vi "FPGA Main High Throughput.vi"() -> ()   [LabVIEW 2019]
doc: "The myRIO v1.2 FPGA Shipping Personality. This personality contains support for:\n- 1 Button\n- 4 LED\n- 4 Analog Input channels with 1 Sample\n- 1 Analog Input channel with N Samples\n- 2 Analog Output channels with 1 Sample\n- 1 Analog Output channel with N Samples\n- 16 Digital I/O channels with 1 Sample\n- 1 Digital Input channel with N Samples\n- 1 Digital Output channel with N Samples"
uses:
  Sub VIs/Utilities/Start Boolean.ctl
  <vilib>/Platform/TimedLoop/XDataNode/timing_clust.ctl
  <vilib>/Platform/TimedLoop/XDataNode/nitl_modes.ctl
  <vilib>/Platform/TimedLoop/XDataNode/wakeup.ctl
  <vilib>/rvi/Emulation/niFpgaGetClockAttributes.vi
  <vilib>/rvi/Emulation/niFpgaSctlEmulationGetInTimedLoop.vi
  <vilib>/rvi/Emulation/niFpgaEmulationReportErrorSimple.vi
  <vilib>/rvi/eio/common/nirviEmuTemplateMethod_errors.vi
  <vilib>/rvi/Emulation/niFpgaProcessEmulError.vi
  <vilib>/rvi/Emulation/niFpgaCriticalErrorInLSC.vi
  <vilib>/rvi/Emulation/niFpgaEmulationIsFPGAContextNoSignature.vi
  <vilib>/rvi/errors/niFpgaSetErrorForExecOnDevCompSimple.vi
  <vilib>/rvi/eio/common/nirviEmuReportErrorAndStop.vi
  <vilib>/rvi/DataTransferAndStorage/Container/Common/niFpgaContainerGetUniqueNameForEmu.vi
  <vilib>/rvi/FIFO/Fifo_Resource/nirvififoEmulationSetSize.vi
  <vilib>/rvi/FIFO/Fifo_Resource/nirviFifoEmulationQueueMgr.vi
  <instcachedir>/0/nirviFifoEmulationQueueMgr_E5CAEC123FF24DC58D834DCA3CDAA9B5.lvgen/nirviFifoEmulationQueueMgr_E5CAEC123FF24DC58D834DCA3CDAA9B5_002.vi
  <vilib>/Utility/error.llb/Clear Errors.vi
  <vilib>/rvi/FIFO/Fifo_Resource/nirvififoEmulationCreateLock.vi
  <vilib>/rvi/FIFO/Fifo_Resource/nirvififoEmulationObtainLock.vi
  <vilib>/rvi/FIFO/Fifo_Resource/nirvififoEmulationReleaseLock.vi
  <vilib>/rvi/occurrence/nirviWaitOnOccurrenceBase.vi
  <vilib>/rvi/errors/nirviReportUnexpectedCaseInternalError.vi
  <vilib>/rvi/errors/nirviReportUnexpectedCaseInternalError (U32).vi
  <vilib>/rvi/FIFO/Fifo_Resource/nirvififoEmulationDetermineInputValidOut.vi
  <vilib>/rvi/interface/RandomDataEmulation/niFpgaRandomDataHandleErrors.vi
  <vilib>/rvi/DataTransferAndStorage/Container/Common/niFpgaContainerSetEmuInfo.vi
  <vilib>/rvi/DataTransferAndStorage/Container/Common/niFpgaContainerExecOnDevCompGetState.vi
  <vilib>/eio/EIONode/EIONode.xnode
  <vilib>/rvi/DataTransferAndStorage/Container/XNode/niFpgaContainer.xnode
  <vilib>/rvi/FIFO/Fifo_Resource/nirvififoEmulationRead.vi
  <vilib>/rvi/FIFO/Fifo_Resource/nirvififoEmulationWrite.vi
  <vilib>/rvi/interface/RandomDataEmulation/nirviRandomDataFpgaReadWriteTemplate.vi
  <vilib>/Platform/TimedLoop/XDataNode/XDataNode.xnode
  <vilib>/rvi/LocalResourceManager/LocalResourceManager.xnode
  <vilib>/rvi/FIFO/Fifo_Resource/niFpgaFifoEmulationRefIn.vi
  <vilib>/Platform/TimedLoop/XDataNode/XDNodeRunTimeDep.lvlib
panel:
  out "AI.B_1.VAL":u16
  out "AI.B_2.VAL":u16
  out "AI.B_3.VAL":u16
  out "AI.B_0.VAL":u16
  in  "AO.B_1.VAL":u16
  in  "AO.B_0.VAL":u16
  out "DIO.B_7:0.IN":u8 format="%08b"
  in  "DIO.B_7:0.DIR":u8 format="%08b"
  in  "DIO.B_7:0.OUT":u8 format="%08b"
  in  "SYS.SELECTB":u8 format="%08b"
  out "DIO.B_15:8.IN":u8 format="%08b"
  in  "DIO.B_15:8.DIR":u8 format="%08b"
  in  "DIO.B_15:8.OUT":u8 format="%08b"
  in  "DO.A_1.IRQ.SELECT":bool
  in  "AO.A_0.IRQ.SELECT":bool
  in  "AO.A_0.VAL":u16
  out "AO.A_0.IDL":bool
  out "AO.SYS.STAT":bool
  in  "AO.SYS.GO":T1
  in  "AO.A_1.VAL":u16
  out "AI.A_0.VAL":u16
  out "AI.A_3.VAL":u16
  out "AI.A_2.VAL":u16
  out "AI.A_1.VAL":u16
  in  "DO.A_1.ClockDivisor":u16 caption="AO LoopRate(Ticks)"
  in  "DI.A_0.ClockDivisor":u16 caption="AO LoopRate(Ticks)"
  out "DO.A_1.IDL":bool
  in  "DI.A_0.ENA":bool
  out "DI.A_0.IDL":bool
  out "DIO.A_15:8.IN":u8 format="%08b"
  in  "DIO.A_15:8.DIR":u8 format="%08b"
  in  "DIO.A_15:8.OUT":u8 format="%08b"
  out "DIO.A_7:0.IN":u8 format="%08b"
  in  "DIO.A_7:0.DIR":u8 format="%08b"
  in  "DIO.A_7:0.OUT":u8 format="%08b"
  out "AI.A_0.IDL":bool
  in  "AI.A_0.SampleRate":u32=40000 caption="Count(Ticks)"
  out "SYS.AI.RDY":bool
  in  "AO.A_0.SampleRate":u32=40000 caption="AO LoopRate(Ticks)"
  out "SYS.RDY":bool
  out "SYS.BLOCK.A/AI0.RDY":bool
  in  "SYS.SELECTA":u8 format="%08b"
  out "DI.BTN":u8 format="%08b"
  in  "DO.LED3:0":u8 format="%04b"
  out "ACC.X.VAL":u16
  out "ACC.Y.VAL":u16
  out "SYS.ACC.RDY":bool
  out "ACC.Z.VAL":u16
  # "System"
  # "Connector B"
  # "Connector A"
  # "Onboard Devices"
  # "Accelerometer"
  # "Analog Input"
  # "Analog Output"
  # "Digital I/O"
  # "Analog Input"
  # "Analog Output"
  # "Digital I/O"
  # "Block Write AO"
  # "Buttons & LEDs"
  # "IO Configuration"
  # "Block Read AI"
  # "Block Read DI"
  # "Block Write DO"
  # "IO Configuration"
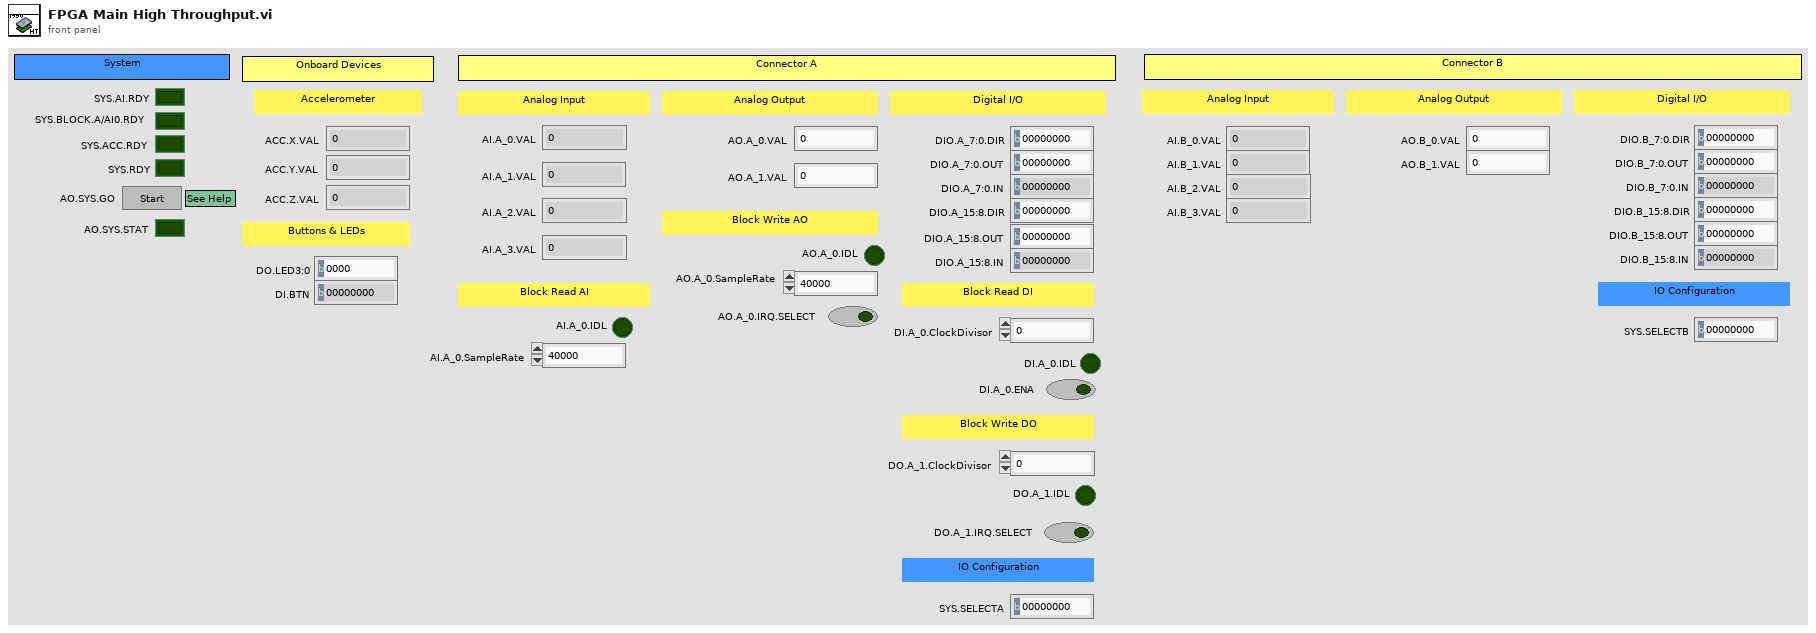
[diagram p1: front panel]
types:
  T1 = typedef "Start Boolean.ctl" = bool
  T2 = typedef "XDNodeRunTimeDep.lvlib/timing_clust.ctl" = cluster{"Expected End [f-1]":u64, "Actual End [f-1]":u64, "Finished Late? [f-1]":bool, "Expected End [i-1]":u64, "Actual End [i-1]":u64, "Finished Late? [i-1]":bool, "Expected Start [i]":u64, "Actual Start [i]":u64, "Expected Start [f]":u64, "Actual Start [f]":u64, "Source Name":string, "Structure Name":string, "Period":i64, "Deadline":i64, "Offset":i64, "Start":i64, "Priority":i32, "Timeout":i32, "Mode":T3, "Wakeup Reason":T4, "Error":errorcluster, "Source Type":string, "Secondary Source Type":string, "Global End Time":u64, "Global Start Time":u64, "Frame Duration":u64, "Iteration Duration":u64, "Assigned CPU":i32, "I/O Scan Engine Mode":u32}
  T3 = typedef "XDNodeRunTimeDep.lvlib/nitl_modes.ctl" = enum32{"No Change", "Process missed periods, maintain original phase", "Discard missed periods, maintain original phase", "Process missed periods, ignore original phase", "Discard missed periods, ignore original phase"}
  T4 = typedef "XDNodeRunTimeDep.lvlib/wakeup.ctl" = enum32{"Normal", "Aborted", "Asynchronous wakeup", "Timing source error", "Timed loop error", "Timeout"}
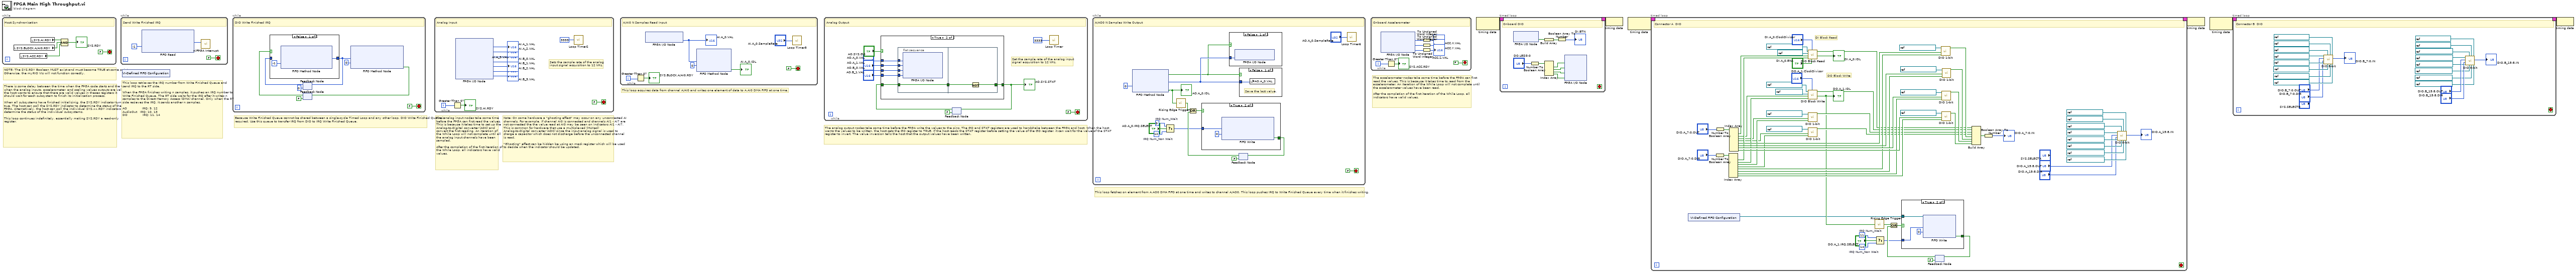
[diagram p0: block diagram]
diagram:
  # "This loop acquires data from channel A/AI0 and writes one element of data to A.AI0 DMA FIFO at one time."
  # "The accelerometer nodes take some time before the FPGA can first read the values. This is because it takes time to read from the accelerometer. An iteration of the While Loop will not complete until the accelerometer values have been read.\n\nAfter the completion of the first iteration of the While Loop, all indicators have valid values."
  # "This loop fetches on element from A.AO0 DMA FIFO at one time and writes to channel A/AO0. This loop pushes IRQ to Write Finished Queue every time when it finishes writing."
  # "The analog output nodes take some time before the FPGA write the values to the pins. The GO and STAT registers are used to handshake between the FPGA and host. When the host wants the values to be written, the host sets the GO register to TRUE. If the host reads the STAT register before setting the value of the GO register, it can wait for the value of the STAT register to invert. The value inversion tells the host that the output values have been written."
  # "The analog input nodes take some time before the FPGA can first read the values. This is because it takes time to set up the Analog-to-Digital converter (ADC) and convert the first reading. An iteration of the While Loop will not complete until all the analog input channels have been sampled.\n\nAfter the completion of the first iteration of the While Loop, all indicators have valid values."
  # "Because Write Finished Queue cannot be shared between a single-cycle Timed Loop and any other loop, DIO Write Finished Queue is required. Use this queue to transfer IRQ from DIO to IRQ Write Finished Queue."
  # "This loop retrieves the IRQ number from Write Finished Queue and send IRQ to the RT side. \n\nWhen the FPGA finishes writing n samples, it pushes an IRQ number to Write Finished Queue. The RT side waits for the IRQ after it writes n samples to the Direct Memory Access (DMA) channel. Only when the RT side recieves the IRQ, it sends another n samples.\n\nAO               IRQ: 9, 12\nAudioOut   IRQ: 10, 13\nDO               IRQ: 11, 14"
  # "NOTE: The SYS.RDY Boolean MUST exist and must become TRUE at some point. Otherwise, the myRIO VIs will not function correctly."
  # "There is some delay between the time when the FPGA code starts and the time when the analog inputs, accelerometer, and scaling values outputs are valid. If the host wants to ensure that there are valid values in theses registers it should wait for each subsystem to finish its initialization process. \n\nWhen all subsystems have finished initializinig, the SYS.RDY indicator turns true. The host can poll the SYS.RDY indicator to determine the status of the FPGA. Alternatively, the host can poll the individual SYS.xx.RDY indicators to determine the status of the individual subsystems.\n\nThis loop continues indefinitely, essentially making SYS.RDY a read-only register."
  # "Note: On some hardware a \"ghosting effect\" may occur on any unconnected AI channels. For example, if channel AI0 is connected and channels AI1 - AI7 are not connected the the value read at AI0 may be seen on indicators AI1 - AI7. This is common for hardware that use a multiplexed (MUXed) Analog-to-Digital converter (ADC) since the input analog signal is used to charge a capacitor which does not discharge before the unconnected channel is read.\n\n\"Ghosting\" effect can be hidden be using an mask register which will be used to decide when the indicator should be updated."
  n1 = while {
    stop <- FALSE stop-if-true
    # "Host Synchronization"
    n2 = local read "SYS.BLOCK.A/AI0.RDY"() -> (w9:bool)
    n3 = local read "SYS.ACC.RDY"() -> (w7:bool)
    n4 = local read "SYS.AI.RDY"() -> (w11:bool)
    n5 = Compound Arithmetic op=AND(w11, w9, w7) -> (→"SYS.RDY":bool)
  }
  n6 = while {
    stop <- FALSE stop-if-true
    # "Send Write Finished IRQ"
    n7 = xnode ("FIFO Read")("Timeout"=-1) -> ("Element"=w14:u8)  [unwired: 1 in, 2 out]
    n8 = call <vilib>:"niFPGA Interrupt.vi"("IRQ Number (0)"=w14) -> ()  [unwired: 2 in]
  }
  n9 = xnode "VI-Defined FIFO Configuration"() -> ()  [unwired: 1 out]
  n10 = while {
    stop <- FALSE stop-if-true
    # "DIO Write Finished IRQ"
    n11 = feedback #1(u8 0 ("Element")) -> (w17:u8)
    n12 = feedback #2(FALSE ("Timed Out?")) -> (w21:bool)
    n13 = case shown="False" w21 {
      tunnel: [w23 w25] -> w18
      tunnel: w17 -> [_ w25]
      frame False {
        n14 = xnode ("FIFO Method Node")("Timeout"=-1) -> ("Element"=w23:u8)  [unwired: 1 in, 2 out]
      }
      frame True {
      }
    }
    n15 = feedback-in #1(w18) -> ()
    n16 = xnode ("FIFO Method Node")("Element"=w18, "Timeout"=0) -> ("Timed Out?"=w19:bool)  [unwired: 1 in, 1 out]
    n17 = feedback-in #2(w19) -> ()
  }
  n18 = while {
    i -> [w30]
    stop <- FALSE stop-if-true
    # "Sets the sample rate of the analog \ninput signal acquisition to 12 kHz."
    # "Analog Input"
    n19 = Greater Than 0?(x=w30) -> (x > 0?=→"SYS.AI.RDY":bool)
    n20 = xnode "FPGA I/O Node"() -> ("ConnectorA/AI1"=→"AI.A_1.VAL":u16, "ConnectorA/AI2"=→"AI.A_2.VAL":u16, "ConnectorA/AI3"=→"AI.A_3.VAL":u16, "ConnectorB/AI0"=→"AI.B_0.VAL":u16, "ConnectorB/AI1"=→"AI.B_1.VAL":u16, "ConnectorB/AI2"=→"AI.B_2.VAL":u16, "ConnectorB/AI3"=→"AI.B_3.VAL":u16)  [unwired: 7 in, 7 out]
    n21 = call "Loop Timer2"("Count(Ticks)"=u32 3333) -> ()  [unwired: 1 out]
  }
  n22 = while {
    i -> [w38]
    stop <- FALSE stop-if-true
    # "A/AI0 N Samples Read Input"
    n23 = Greater Than 0?(x=w38) -> (x > 0?=→"SYS.BLOCK.A/AI0.RDY":bool)
    n24 = xnode "FPGA I/O Node"() -> ("ConnectorA/AI0"=w39:u16)  [unwired: 1 in, 1 out]
    "AI.A_0.VAL" <- w39
    n25 = xnode ("FIFO Method Node")("Element"=w39, "Timeout"=0) -> ("Timed Out?"=→"AI.A_0.IDL":bool)  [unwired: 1 in, 1 out]
    n26 = call "Loop Timer5"("Count(Ticks)"="AI.A_0.SampleRate") -> ()  [unwired: 1 out]
  }
  n27 = while {
    stop <- FALSE stop-if-true
    # "Set the sample rate of the analog input \nsignal acquisition to 12 kHz."
    # "Analog Output"
    n28 = feedback #3(FALSE) -> (w50:bool)
    n29 = case shown="True" "AO.SYS.GO" {
      tunnel: "AO.A_0.VAL" -> [_ w61]
      tunnel: "AO.A_1.VAL" -> [_ w60]
      tunnel: w50 -> [w54 w59]
      tunnel: [w54 w57] -> w49
      tunnel: "AO.B_0.VAL" -> [_ w56]
      tunnel: "AO.B_1.VAL" -> [_ w55]
      frame False {
      }
      frame True {
        n30 = flat-sequence {
          tunnel: w61 -> [w66]
          tunnel: w60 -> [w65]
          tunnel: w59 -> [w64]
          tunnel: [w64] -> w58
          tunnel: w56 -> [w63]
          tunnel: w55 -> [w62]
          tunnel: w58 -> [w68]
          tunnel: [w67] -> w57
          frame #0 {
            n31 = xnode "FPGA I/O Node"("ConnectorA/AO0"=w66, "ConnectorA/AO1"=w65, "ConnectorB/AO0"=w63, "ConnectorB/AO1"=w62) -> ()  [unwired: 4 in, 4 out]
          }
          frame #1 {
            n32 = Not(x=w68) -> (.not. x?=w67:bool)
          }
        }
      }
    }
    "AO.SYS.STAT" <- w49
    n33 = feedback-in #3(w49) -> ()
    n34 = call "Loop Timer"("Count(Ticks)"=u32 3333) -> ()  [unwired: 1 out]
  }
  n35 = while {
    stop <- FALSE stop-if-true
    w72 = u8 12  # IRQ Num_Non Wait
    w70 = u8 9  # IRQ Num_Wait
    # "A/AO0 N Samples Write Output"
    n36 = xnode ("FIFO Method Node")("Timeout"=0) -> ("Element"=w80:u16, "Timed Out?"=w78:bool)  [unwired: 1 in, 1 out]
    "AO.A_0.IDL" <- w78
    n37 = Select(t=w70, s="AO.A_0.IRQ.SELECT", f=w72) -> (s? t:f=w69:u8)
    n38 = call "Rising Edge Trigger.vi"("Signal"=w78) -> ("Trigger?"=w73:bool)
    n39 = case shown="False" w78 {
      tunnel: w80 -> [w87 _]
      frame False {
        n40 = xnode "FPGA I/O Node"("ConnectorA/AO0"=w87) -> ()  [unwired: 1 in, 1 out]
      }
      frame True {
      }
    }
    n41 = feedback #4(FALSE ("Timed Out?")) -> (w74:bool)
    n42 = Or(x=w73, y=w74) -> (x .or. y?=w76:bool)
    n43 = case shown="True" w76 {
      selector: w76 -> [w83 _]
      tunnel: [w83 w86] -> w75
      tunnel: w69 -> [_ w84]
      frame False {
      }
      frame True {
        n44 = xnode ("FIFO Write")("Element"=w84, "Timeout"=0) -> ("Timed Out?"=w86:bool)  [unwired: 1 in, 1 out]
      }
    }
    n45 = feedback-in #4(w75) -> ()
    n46 = case shown="False" w78 {
      tunnel: w80 -> [w88 _]
      frame False {
        # "Save the last value."
        n47 = local write "AO.A_0.VAL"(w88) -> ()
      }
      frame True {
      }
    }
    n48 = call "Loop Timer6"("Count(Ticks)"="AO.A_0.SampleRate") -> ()  [unwired: 1 out]
  }
  n49 = while {
    i -> [w93]
    stop <- FALSE stop-if-true
    # "Onboard Accelerometer"
    n50 = xnode "FPGA I/O Node"() -> ("AccelerationX"=w96:i16, "AccelerationY"=w95:i16, "AccelerationZ"=w94:i16)  [unwired: 3 in, 3 out]
    n51 = Greater Than 0?(x=w93) -> (x > 0?=→"SYS.ACC.RDY":bool)
    n52 = To Unsigned Word Integer(number=w96) -> (unsigned 16bit integer=→"ACC.X.VAL":u16)
    n53 = To Unsigned Word Integer(number=w95) -> (unsigned 16bit integer=→"ACC.Y.VAL":u16)
    n54 = To Unsigned Word Integer(number=w94) -> (unsigned 16bit integer=→"ACC.Z.VAL":u16)
  }
  n55 = node-c288() -> (w4:T2)  [unwired: 1 in]
  n56 = timed-loop {
    timing: w4 -> [_]
    timing-out: [_] -> w3
    stop <- _ stop-if-true
    # "Onboard DIO"
    n57 = xnode "FPGA I/O Node"() -> ("Button0"=w106:bool)  [unwired: 1 in, 1 out]
    n58 = Number To Boolean Array(number="DO.LED3:0") -> (Boolean array=w102:bool[])
    n59 = Build Array(w106) -> (w105:bool[])
    n60 = Index Array(array=w102) -> (element #1=w101:bool, element #2=w100:bool, element #3=w99:bool, element #4=w98:bool)  [unwired: 4 in]
    n61 = Boolean Array To Number(Boolean array=w105) -> (number=→"DI.BTN":u8)
    n62 = xnode "FPGA I/O Node"("LED0"=w101, "LED1"=w100, "LED2"=w99, "LED3"=w98) -> ()  [unwired: 4 in, 4 out]
  }
  n63 = node-c288(w3) -> ()
  n64 = node-c288() -> (w6:T2)  [unwired: 1 in]
  n65 = timed-loop {
    timing: w6 -> [_]
    timing-out: [_] -> w5
    stop <- _ stop-if-true
    w112 = u8 14  # IRQ Num_Non Wait
    w113 = u8 11  # IRQ Num_Wait
    # "DO Block Write"
    # "DI Block Read"
    # "Connector A  DIO"
    n66 = xnode "VI-Defined FIFO Configuration"() -> ("FIFO Out"=w109:refnum<k21>)
    n67 = Number To Boolean Array(number="DIO.A_7:0.DIR") -> (Boolean array=w154:bool[])
    n68 = Number To Boolean Array(number="DIO.A_7:0.OUT") -> (Boolean array=w160:bool[])
    n69 = Index Array(array=w154) -> (element #1=w137:bool, element #2=w135:bool, element #3=w132:bool, element #4=w130:bool, element #5=w153:bool, element #6=w152:bool, element #7=w151:bool, element #8=w150:bool)  [unwired: 8 in]
    n70 = Index Array(array=w160) -> (element #1=w139:bool, element #2=w136:bool, element #3=w133:bool, element #4=w131:bool, element #5=w158:bool, element #6=w157:bool, element #7=w156:bool, element #8=w155:bool)  [unwired: 8 in]
    n71 = call "DIO 1-bit.vi"("DIR"=w132, "OUT"=w133, "DIO Refnum"=refnum<k21> "ConnectorA/DIO2") -> ("IN"=w129:bool)  [unwired: 8 in]
    n72 = call "DIO Block Read.vi"("ENA"="DI.A_0.ENA", "Divisor"="DI.A_0.ClockDivisor", "DIR"=w137, "OUT"=w139, "FIFO In"=refnum<k21> "A.DI0 DMA", "DIO Refnum"=refnum<k21> "ConnectorA/DIO0" ("DIO.0/QE.A")) -> ("Timed Out?"=→"DI.A_0.IDL":bool, "IN"=w138:bool)  [unwired: 4 in]
    n73 = call "DIO Block Write.vi"("Divisor"="DO.A_1.ClockDivisor", "DIR"=w135, "OUT"=w136, "DMA FIFO In"=refnum<k21> "A.DO1 DMA", "DIO Refnum"=refnum<k21> "ConnectorA/DIO1" ("DIO.1/QE.B")) -> ("Timed Out?"=w110:bool, "IN"=w134:bool)  [unwired: 5 in]
    "DO.A_1.IDL" <- w110
    n74 = call "DIO 1-bit.vi"("DIR"=w130, "OUT"=w131, "DIO Refnum"=refnum<k21> "ConnectorA/DIO3" ("DIO/PWM")) -> ("IN"=w128:bool)  [unwired: 8 in]
    n75 = call "Rising Edge Trigger.vi"("Signal"=w110) -> ("Trigger?"=w116:bool)
    n76 = Select(t=w113, s="DO.A_1.IRQ.SELECT", f=w112) -> (s? t:f=w111:u8)
    n77 = feedback #5(FALSE ("Timed Out?")) -> (w117:bool)
    n78 = Or(x=w116, y=w117) -> (x .or. y?=w118:bool)
    n79 = case shown="True" w118 {
      selector: w118 -> [w175 _]
      tunnel: [w175 w177] -> w115
      tunnel: w109 -> [_ w178]
      tunnel: w111 -> [_ w176]
      frame False {
      }
      frame True {
        n80 = xnode ("FIFO Write")("Element"=w176, "Timeout"=0, "FIFO In"=w178) -> ("Timed Out?"=w177:bool)  [unwired: 1 out]
      }
    }
    n81 = feedback-in #5(w115) -> ()
    n82 = call "DIO 1-bit.vi"("DIR"=w153, "OUT"=w158, "DIO Refnum"=refnum<k21> "ConnectorA/DIO4" ("DIO.0/QE.A")) -> ("IN"=w149:bool)  [unwired: 8 in]
    n83 = call "DIO 1-bit.vi"("DIR"=w151, "OUT"=w156, "DIO Refnum"=refnum<k21> "ConnectorA/DIO6") -> ("IN"=w147:bool)  [unwired: 8 in]
    n84 = call "DIO 1-bit.vi"("DIR"=w150, "OUT"=w155, "DIO Refnum"=refnum<k21> "ConnectorA/DIO7" ("DIO/PWM")) -> ("IN"=w146:bool)  [unwired: 8 in]
    n85 = call "DIO 1-bit.vi"("DIR"=w152, "OUT"=w157, "DIO Refnum"=refnum<k21> "ConnectorA/DIO5" ("DIO.1/QE.B")) -> ("IN"=w148:bool)  [unwired: 8 in]
    n86 = Build Array(w138, w134, w129, w128, w149, w148, w147, w146) -> (w145:bool[])
    n87 = Boolean Array To Number(Boolean array=w145) -> (number=→"DIO.A_7:0.IN":u8)
    n88 = call "DIO 8-bit.vi"("DIO 7 Refnum"=refnum<k21> "ConnectorA/DIO15" ("DIO.1/I2C.SCL"), "DIO 0 Refnum"=refnum<k21> "ConnectorA/DIO8" ("DIO/PWM"), "DIO 6 Refnum"=refnum<k21> "ConnectorA/DIO14" ("DIO.0/I2C.SDA"), "DIO 1 Refnum"=refnum<k21> "ConnectorA/DIO9" ("DIO/PWM"), "DIO 5 Refnum"=refnum<k21> "ConnectorA/DIO13" ("DIO Refnum"), "DIO 2 Refnum"=refnum<k21> "ConnectorA/DIO10" ("DIO/PWM"), "DIO 4 Refnum"=refnum<k21> "ConnectorA/DIO12" ("DIO.1/QE.B"), "DIR 7:0"="DIO.A_15:8.DIR", "OUT 7:0"="DIO.A_15:8.OUT", "DIO 3 Refnum"=refnum<k21> "ConnectorA/DIO11" ("DIO.0/QE.A")) -> ("IN 7:0"=→"DIO.A_15:8.IN":u8)  [unwired: 1 in]
  }
  n89 = node-c288(w5) -> ()
  n90 = node-c288() -> (w2:T2)  [unwired: 1 in]
  n91 = timed-loop {
    timing: w2 -> [_]
    timing-out: [_] -> w1
    stop <- _ stop-if-true
    # "Connector B  DIO"
    n92 = call "DIO 8-bit.vi"("DIO 7 Refnum"=refnum<k21> "ConnectorB/DIO7" ("DIO.2/SPI.SCLK"), "DIO 0 Refnum"=refnum<k21> "ConnectorB/DIO0" ("DIO0 Refnum"), "DIO 6 Refnum"=refnum<k21> "ConnectorB/DIO6" ("DIO.1/SPI.MOSI"), "DIO 1 Refnum"=refnum<k21> "ConnectorB/DIO1" ("DIO1 Refnum"), "DIO 5 Refnum"=refnum<k21> "ConnectorB/DIO5" ("DIO.0/SPI.MISO"), "DIO 2 Refnum"=refnum<k21> "ConnectorB/DIO2" ("DIO2 Refnum"), "DIO 4 Refnum"=refnum<k21> "ConnectorB/DIO4" ("DIO Refnum"), "DIR 7:0"="DIO.B_7:0.DIR", "OUT 7:0"="DIO.B_7:0.OUT", "DIO 3 Refnum"=refnum<k21> "ConnectorB/DIO3" ("DIO3 Refnum")) -> ("IN 7:0"=→"DIO.B_7:0.IN":u8)  [unwired: 1 in]
    n93 = call "DIO 8-bit.vi"("DIO 7 Refnum"=refnum<k21> "ConnectorB/DIO15" ("DIO.2/SPI.SCLK"), "DIO 0 Refnum"=refnum<k21> "ConnectorB/DIO8" ("DIO0 Refnum"), "DIO 6 Refnum"=refnum<k21> "ConnectorB/DIO14" ("DIO.1/SPI.MOSI"), "DIO 1 Refnum"=refnum<k21> "ConnectorB/DIO9" ("DIO1 Refnum"), "DIO 5 Refnum"=refnum<k21> "ConnectorB/DIO13" ("DIO.0/SPI.MISO"), "DIO 2 Refnum"=refnum<k21> "ConnectorB/DIO10" ("DIO2 Refnum"), "DIO 4 Refnum"=refnum<k21> "ConnectorB/DIO12" ("DIO Refnum"), "DIR 7:0"="DIO.B_15:8.DIR", "OUT 7:0"="DIO.B_15:8.OUT", "DIO 3 Refnum"=refnum<k21> "ConnectorB/DIO11" ("DIO3 Refnum")) -> ("IN 7:0"=→"DIO.B_15:8.IN":u8)  [unwired: 1 in]
  }
  n94 = node-c288(w1) -> ()
